vi "gun_speed_override_datastore.vi"(9 "Mode":enum16{"Process OVR", "Reset OVR", "Set OVR"}(ring), 10 "Control Type":T1, 11 "Control Input":dbl) -> (1 "OVR mode":enum16{"Normal", "Override"}(ring), 2 "Control Type Output":T1, 3 "Control Output":dbl)   [LabVIEW 2011]
uses:
  gun_motor_state.ctl
panel:
  in  "max_dist":dbl=20.0
  in  "max_speed":dbl=217.0
  in  "Gain":dbl[](array[numeric])=[0.047, 7.0, 0.67, 0.0]
  # "pow\n\nspeed\n\ndist\n\noff"
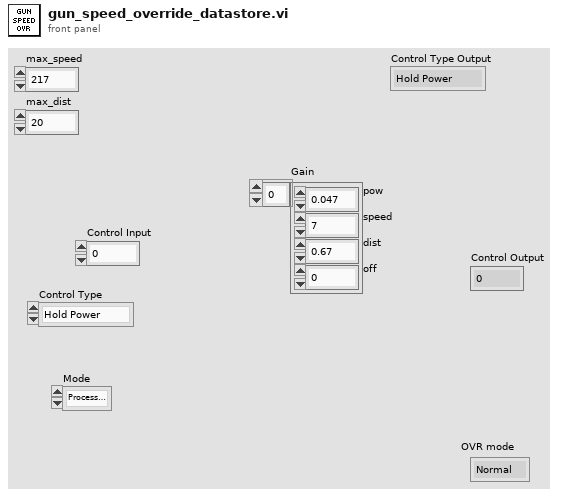
[diagram p1: front panel]
types:
  T1 = typedef "gun_motor_state.ctl" = enum16{"Hold Power", "Hold Speed", "Hold Distance", "Stop"}
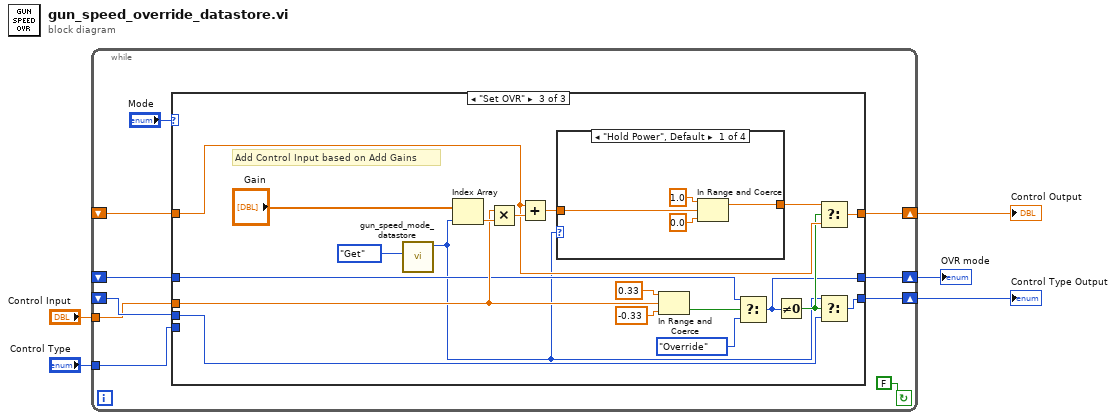
[diagram p0: block diagram]
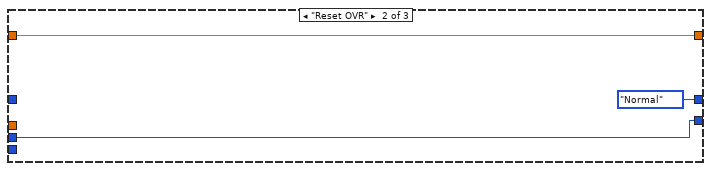
[diagram p4: hidden frame]
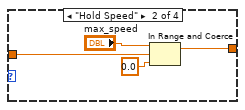
[diagram p5: hidden frame]
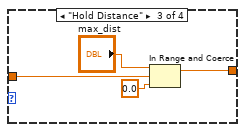
[diagram p6: hidden frame]
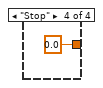
[diagram p7: hidden frame]
diagram:
  n1 = while {
    shift-right: [w11] -> w5
    shift-left: _ -> [w10]
    shift-right: [w13] -> w4
    shift-left: _ -> [w12]
    shift-right: [w14] -> w3
    shift-left: _ -> [w9]
    tunnel: "Control Input" -> [w8]
    tunnel: "Control Type" -> [w7]
    stop <- FALSE continue-if-true
    n2 = case shown="\"Set OVR\"" "Mode" {
      tunnel: [w22 enum16{"Normal", "Override"}."Normal" ("OVR mode") w37] -> w14
      tunnel: [w19 w31 w36] -> w13
      tunnel: w12 -> [w18 w31 w45]
      tunnel: [w21 w30 w47] -> w11
      tunnel: w10 -> [w20 w30 w46]
      tunnel: w9 -> [w23 _ w39]
      tunnel: w8 -> [w17 _ w43]
      tunnel: w7 -> [w16 _ _]
      frame "Process OVR", Default {
        n3 = case shown="\"Normal\", Default" w23 {
          selector: w23 -> [w24 w29]
          tunnel: [w24 w29] -> w22
          tunnel: [w26 w28] -> w21
          tunnel: w20 -> [_ w28]
          tunnel: [w25 w27] -> w19
          tunnel: w18 -> [_ w27]
          tunnel: w17 -> [w26 _]
          tunnel: w16 -> [w25 _]
          frame "Normal", Default {
            # "Store Current Data"
          }
          frame "Override" {
            # "Return OVR data"
          }
        }
      }
      frame "Reset OVR" {
      }
      frame "Set OVR" {
        # "Add Control Input based on Add Gains"
        n4 = call "gun_speed_mode_datastore.vi"("data_store_mode"=enum16{"Set", "Get"}."Get") -> ("Shooter Control Mode Out"=w33:T1)  [unwired: 10 in]
        n5 = Index Array(array="Gain", index=w33) -> (element=w49:dbl)
        n6 = Multiply(x=w43, y=w49) -> (x*y=w48:dbl)
        n7 = Add(x=w46, y=w48) -> (x+y=w35:dbl)
        n8 = case shown="\"Hold Power\", Default" w33 {
          tunnel: w35 -> [w53 w59 w63 _]
          tunnel: [w52 w58 w60 0.0 ("max_dist")] -> w34
          frame "Hold Power", Default {
            n9 = In Range and Coerce(upper limit=1.0, x=w53, lower limit=0.0) -> (coerced(x)=w52:dbl)  [unwired: 1 out]
          }
          frame "Hold Speed" {
            n10 = In Range and Coerce(upper limit="max_speed", x=w59, lower limit=0.0) -> (coerced(x)=w58:dbl)  [unwired: 1 out]
          }
          frame "Hold Distance" {
            n11 = In Range and Coerce(upper limit="max_dist", x=w63, lower limit=0.0) -> (coerced(x)=w60:dbl)  [unwired: 1 out]
          }
          frame "Stop" {
          }
        }
        n12 = In Range and Coerce(upper limit=0.33, x=w43, lower limit=-0.33) -> (In Range?=w40:bool)  [unwired: 1 out]
        n13 = Select(t=w39, s=w40, f=enum16{"Normal", "Override"}."Override") -> (s? t:f=w37:enum16{"Normal", "Override"})
        n14 = Not Equal To 0?(x=w37) -> (x != 0?=w44:bool)
        n15 = Select(t=w34, s=w44, f=w46) -> (s? t:f=w47:dbl)
        n16 = Select(t=w33, s=w44, f=w45) -> (s? t:f=w36:T1)
      }
    }
  }
  "Control Output" <- w5
  "OVR mode" <- w3
  "Control Type Output" <- w4
